vi "setPropertyObjectValue.vi"(8 "error in (no error)":errorcluster, 9 "Value in":refnum<class "IPropertyObject.lvclass">, 10 "Property Name in":string, 11 "IPropertyObject in":refnum<class "IPropertyObject.lvclass">) -> (0 "error out":errorcluster, 1 "Value out":refnum<class "IPropertyObject.lvclass">, 2 "Property Name out":string, 3 "IPropertyObject out":refnum<class "IPropertyObject.lvclass">)   [LabVIEW 2022 SP3, in "openDAQ.lvlib" / "IBaseObject.lvlib" / "IPropertyObject.lvlib" / "IPropertyObject.lvclass"]
uses:
  <instrlib>/openDAQ/Public/Classes/IPropertyObject/IPropertyObject.lvclass
  C:/Program Files (x86)/National Instruments/LabVIEW 2022/instr.lib/openDAQ/Public/Classes/IBaseObject/IBaseObject.lvclass
  <instrlib>/openDAQ/Public/Classes/IBaseObject/IBaseObject.lvclass/IBaseObject.ctl
  <instrlib>/openDAQ/Public/Classes/IBaseObject/Accessor/Read reference.vi
  <instrlib>/openDAQ/Public/Classes/IBaseObject/Accessor/Write reference.vi
  <instrlib>/openDAQ/Public/Classes/daqCoreTypes/IString/IString.lvclass
  <instrlib>/openDAQ/Binaries/Windows/x86/copendaq32.dll
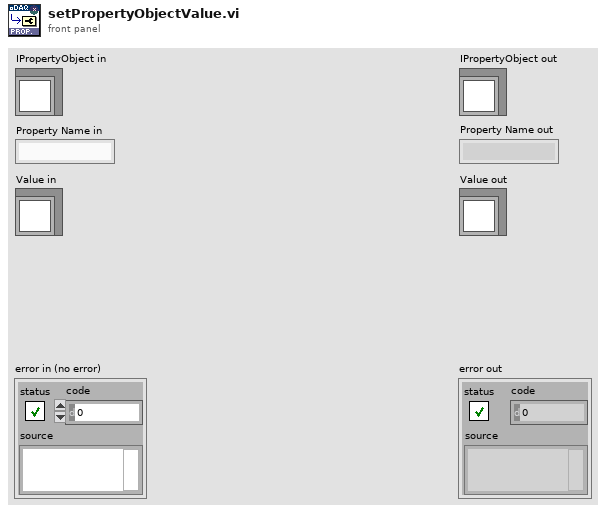
[diagram p1: front panel]
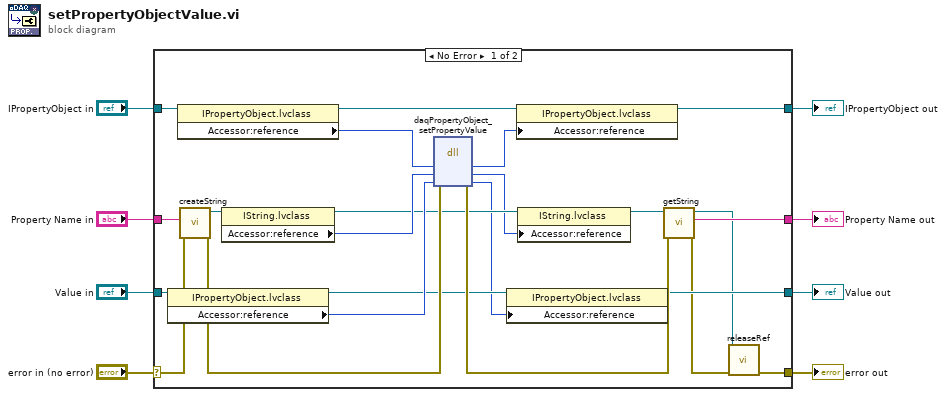
[diagram p0: block diagram]
diagram:
  n1 = case shown="No Error" "error in (no error)" {
    selector: "error in (no error)" -> [w24 w35]
    tunnel: [w12 w35] -> w7
    tunnel: [w26 w34] -> w5
    tunnel: "IPropertyObject in" -> [w29 w34]
    tunnel: "Property Name in" -> [w22 w32]
    tunnel: "Value in" -> [w21 w33]
    tunnel: [w18 w33] -> w1
    tunnel: [w14 w32] -> w3
    frame No Error {
      n2 = property class="IPropertyObject.lvclass"(reference=w21) -> (reference out=w19:refnum<class "IPropertyObject.lvclass">, "Accessor:reference"=w31:i64)  [unwired: 1 in, 1 out]
      n3 = property class="IPropertyObject.lvclass"(reference=w29) -> (reference out=w27:refnum<class "IPropertyObject.lvclass">, "Accessor:reference"=w28:i64)  [unwired: 1 in, 1 out]
      n4 = call <instrlib>:"createString.vi"("error in (no error)"=w24, "String"=w22) -> ("error out"=w23:errorcluster, "IString out"=w20:refnum<class "IString.lvclass">)  [unwired: 8 in]
      n5 = property class="IString.lvclass"(reference=w20) -> (reference out=w16:refnum<class "IString.lvclass">, "Accessor:reference"=w17:i64)  [unwired: 1 in, 1 out]
      n6 = dll-call lib="C:/Program Files (x86)/National Instruments/LabVIEW 2022/instr.lib/openDAQ/Binaries/Windows/x86/copendaq*.*" fn="daqPropertyObject_setPropertyValue"(error in=w23, "config"=w28, "propertyName"=w17, "value"=w31) -> (error out=w30:errorcluster, "config"=w25:i64, "propertyName"=w10:i64, "value"=w9:i64)  [unwired: 3 in, 1 out]
      n7 = property class="IPropertyObject.lvclass"(reference=w19, "Accessor:reference"=w9) -> (reference out=w18:refnum<class "IPropertyObject.lvclass">)  [unwired: 1 in, 1 out]
      n8 = property class="IPropertyObject.lvclass"(reference=w27, "Accessor:reference"=w25) -> (reference out=w26:refnum<class "IPropertyObject.lvclass">)  [unwired: 1 in, 1 out]
      n9 = property class="IString.lvclass"(reference=w16, "Accessor:reference"=w10) -> (reference out=w15:refnum<class "IString.lvclass">)  [unwired: 1 in, 1 out]
      n10 = call <instrlib>:"getString.vi"("error in (no error)"=w30, "IString in"=w15) -> ("error out"=w13:errorcluster, "String out"=w14:string, "IString out"=w11:refnum<class "IString.lvclass">)  [unwired: 7 in]
      n11 = call-dynamic "releaseRef.vi"("error in (no error)"=w13, "IBaseObject in"=w11) -> ("error out"=w12:errorcluster)  [unwired: 9 in]
    }
    frame Error {
    }
  }
  "error out" <- w7
  "IPropertyObject out" <- w5
  "Property Name out" <- w3
  "Value out" <- w1
